vi "USB.vi"() -> ()   [LabVIEW 2019]
panel:
  in  "file no.":u32
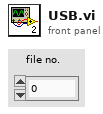
[diagram p1: front panel]
types:
  T1 = enum16{"open", "replace", "create", "open or create", "replace or create", "replace or create with confirmation"}
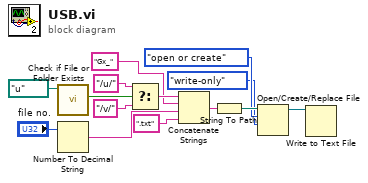
[diagram p0: block diagram]
diagram:
  n1 = call <vilib>:"Check if File or Folder Exists.vi"("path"=path "u:/") -> ("file or folder exists?"=w11:bool)  [unwired: 8 in, 2 out]
  n2 = Number To Decimal String(number="file no.") -> (decimal integer string=w4:string)  [unwired: 1 in]
  n3 = Select(t="/u/", s=w11, f="/v/") -> (s? t:f=w9:string)
  n4 = Concatenate Strings(w9, "Gx_" ("string"), w4, ".txt" ("string")) -> (w8:string)
  n5 = String To Path(string=w8) -> (path=w10:path)
  n6 = Open/Create/Replace File(file path (use dialog)=w10, operation (0:open)=T1."open or create", access (0:read/write)=enum16{"read/write", "read-only", "write-only"}."write-only") -> (refnum out=w1:refnum<file>)  [unwired: 3 in, 2 out]
  n7 = Write to Text File(file (use dialog)=w1) -> ()  [unwired: 3 in, 3 out]
